vi "LS330_Read_Heater.vi"(8 "error in":errorcluster, 10 "Heater":string(combo)="1", 11 "VISA resource name":refnum<visa-resource-name>) -> (0 "error out":errorcluster, 2 "Heater %":dbl, 3 "VISA resource name out":refnum<visa-resource-name>)   [LabVIEW 2021]
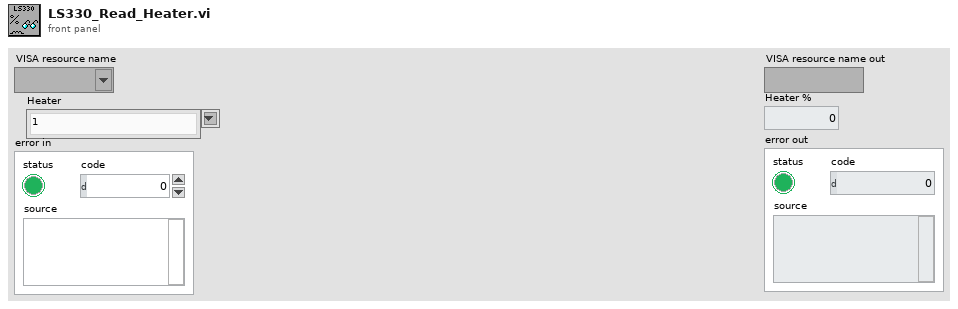
[diagram p1: front panel]
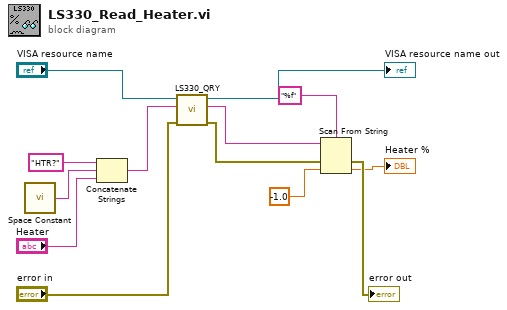
[diagram p0: block diagram]
diagram:
  n1 = call <vilib>:"Space Constant.vi"() -> ("String"=w11:string)
  n2 = Concatenate Strings("HTR?" ("string"), w11, "Heater") -> (w9:string)
  n3 = call "LS330_QRY.vi"("error in"="error in", "CMD"=w9, "VISA resource name"="VISA resource name") -> ("error out"=w4:errorcluster, "OUT"=w5:string, "VISA resource name out"=→"VISA resource name out":refnum<visa-resource-name>)  [unwired: 5 in, 1 out]
  n4 = Scan From String(format string="%f", input string=w5, error in=w4, default 1=-1.0 ("default value 1")) -> (error out=→"error out":errorcluster, output 1=→"Heater %":dbl)  [unwired: 1 in, 2 out]
